vi "Abort Acquisition.vi"(8 "error in (no error)":errorcluster {"code" format="%.0x"}, 10 "Channel Name (1)":string="1", 11 "VISA resource name":refnum<visa-resource-name>) -> (0 "error out":errorcluster {"code" format="%.0x"}, 3 "VISA resource name out":refnum<visa-resource-name>)   [LabVIEW 2014, in "Agilent N6700 Series.lvlib"]
doc: "Aborts an acquisition and returns the DC Power supply to the Idle state. It also resets the WTG-meas bit in the Condition Status register. You initiate an acquisition with the <B>Initiate Acquisition.vi</B>.\n\n<b>Note:</b>\n(1) Do not abort individual channels.\n(2) This VI can generate an error with double modules.\n(3) This VI requires Option 054 (High-Speed Test Extension) to be installed on models N673xA, N674xA, N675xA and N677xA."
uses:
  Agilent N6700 Series.lvlib
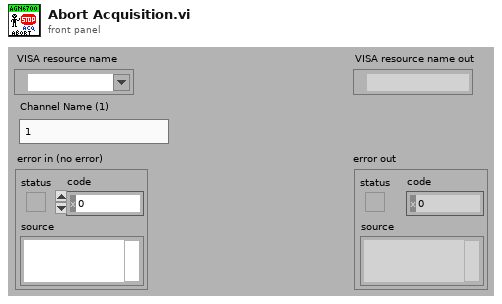
[diagram p1: front panel]
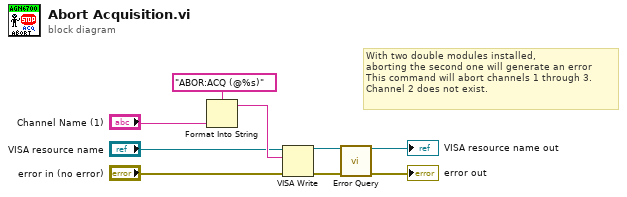
[diagram p0: block diagram]
diagram:
  # "With two double modules installed, \naborting the second one will generate an error \nThis command will abort channels 1 through 3. \nChannel 2 does not exist."
  n1 = Format Into String(format string="ABOR:ACQ (@%s)", "Channel Name (1)") -> (resulting string=w9:string)  [unwired: 2 in, 1 out]
  n2 = VISA Write(VISA resource name="VISA resource name", write buffer=w9, error in (no error)="error in (no error)") -> (VISA resource name out=w2:refnum<visa-resource-name>, error out=w1:errorcluster)  [unwired: 1 out]
  n3 = call "Error Query.vi"("VISA resource name"=w2, "error in (no error)"=w1) -> ("VISA resource name out"=→"VISA resource name out":refnum<visa-resource-name>, "error out"=→"error out":errorcluster)  [unwired: 10 in, 2 out]
